vi "caselar.vi"() -> ()   [LabVIEW 2015]
panel:
  out "String":string
  in  "string 2":string
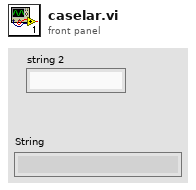
[diagram p1: front panel]
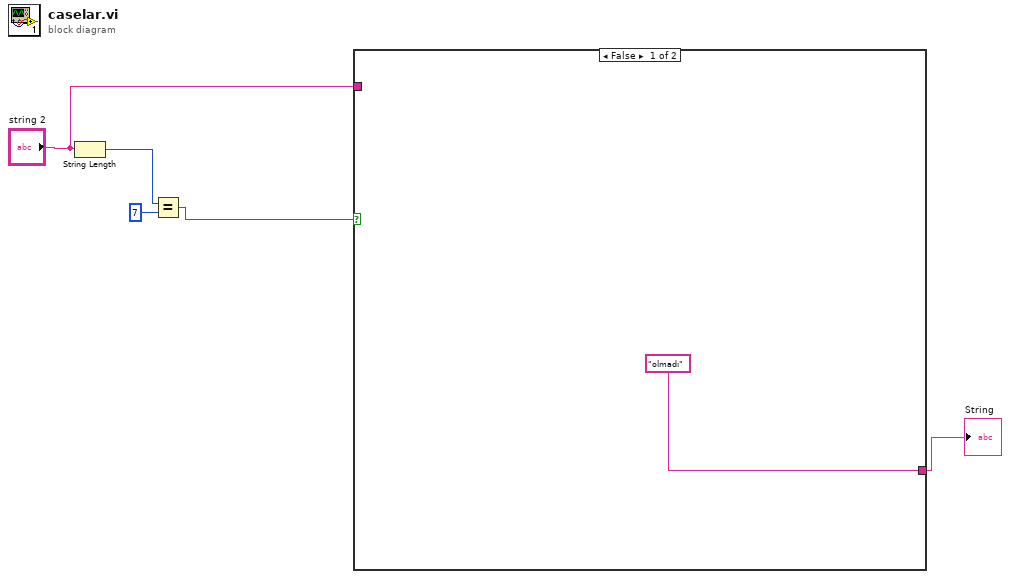
[diagram p0: block diagram]
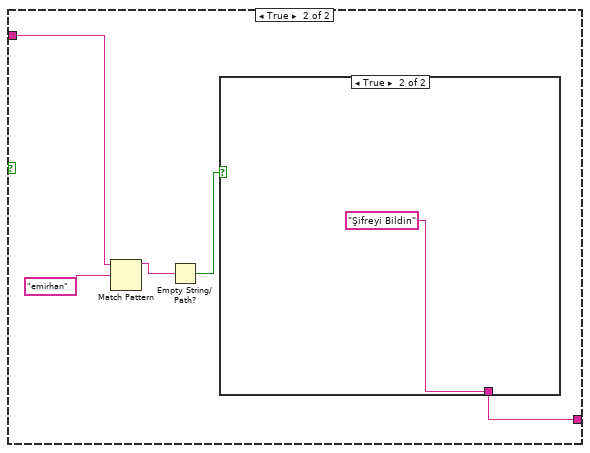
[diagram p2: hidden frame]
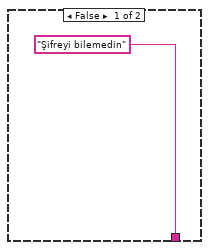
[diagram p3: hidden frame]
diagram:
  n1 = String Length(string="string 2") -> (length=w5:i32)
  n2 = Equal?(x=w5, y=7) -> (x = y?=w4:bool)
  n3 = case shown="False" w4 {
    tunnel: "string 2" -> [_ w10]
    tunnel: ["olmadı" w7] -> w1
    frame False {
    }
    frame True {
      n4 = Match Pattern(string=w10, regular expression="emirhan") -> (before substring=w9:string)  [unwired: 1 in, 3 out]
      n5 = Empty String/Path?(string/path=w9) -> (empty?=w8:bool)
      n6 = case shown="True" w8 {
        tunnel: ["Şifreyi bilemedin" "Şifreyi Bildin"] -> w7
        frame False {
        }
        frame True {
        }
      }
    }
  }
  "String" <- w1
